vi "SPI_CY_target.vi"() -> ()   [LabVIEW 2018]
uses:
  <vilib>/Platform/TimedLoop/XDataNode/timing_clust.ctl
  <vilib>/Platform/TimedLoop/XDataNode/nitl_modes.ctl
  <vilib>/Platform/TimedLoop/XDataNode/wakeup.ctl
  <vilib>/rvi/Emulation/niFpgaGetClockAttributes.vi
  <vilib>/rvi/Emulation/niFpgaSctlEmulationGetInTimedLoop.vi
  <vilib>/rvi/Emulation/niFpgaEmulationReportErrorSimple.vi
  <vilib>/rvi/eio/common/nirviEmuTemplateMethod_errors.vi
  <vilib>/rvi/Emulation/niFpgaCriticalErrorInLSC.vi
  <vilib>/rvi/Emulation/niFpgaProcessEmulError.vi
  <vilib>/rvi/interface/RandomDataEmulation/niFpgaRandomDataHandleErrors.vi
  <vilib>/eio/EIONode/EIONode.xnode
  <vilib>/Platform/TimedLoop/XDataNode/XDataNode.xnode
  <vilib>/rvi/DataTransferAndStorage/Container/XNode/niFpgaContainer.xnode
  <vilib>/rvi/interface/RandomDataEmulation/nirviRandomDataFpgaReadWriteTemplate.vi
  <vilib>/Platform/TimedLoop/XDataNode/XDNodeRunTimeDep.lvlib
panel:
  out "Addr Read":u32
  out "WriteError":bool
  out "Addr":u32
  out "WriteChipComplete":bool
  in  "i":i32
  in  "Parts":i32
  in  "ReadDelay":u8
  in  "Stop":bool
  in  "ReadWords":u32
  in  "NextPart":bool
  out "ReadChipComplete":bool
  in  "Source Name":refnum<k21>="20MHz"
  in  "SelectOperation":enum16{"Read", "Write"}(ring)
  in  "OperationComplete":bool
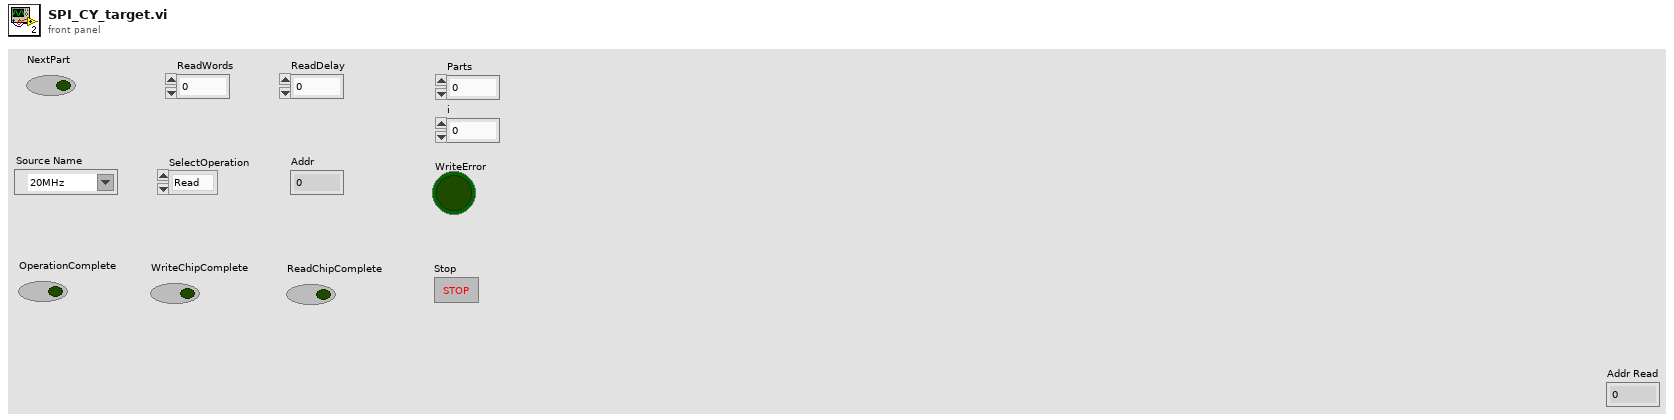
[diagram p1: front panel]
types:
  T1 = typedef "XDNodeRunTimeDep.lvlib/timing_clust.ctl" = cluster{"Expected End [f-1]":u64, "Actual End [f-1]":u64, "Finished Late? [f-1]":bool, "Expected End [i-1]":u64, "Actual End [i-1]":u64, "Finished Late? [i-1]":bool, "Expected Start [i]":u64, "Actual Start [i]":u64, "Expected Start [f]":u64, "Actual Start [f]":u64, "Source Name":string, "Structure Name":string, "Period":i64, "Deadline":i64, "Offset":i64, "Start":i64, "Priority":i32, "Timeout":i32, "Mode":T2, "Wakeup Reason":T3, "Error":errorcluster, "Source Type":string, "Secondary Source Type":string, "Global End Time":u64, "Global Start Time":u64, "Frame Duration":u64, "Iteration Duration":u64, "Assigned CPU":i32, "I/O Scan Engine Mode":u32}
  T2 = typedef "XDNodeRunTimeDep.lvlib/nitl_modes.ctl" = enum32{"No Change", "Process missed periods, maintain original phase", "Discard missed periods, maintain original phase", "Process missed periods, ignore original phase", "Discard missed periods, ignore original phase"}
  T3 = typedef "XDNodeRunTimeDep.lvlib/wakeup.ctl" = enum32{"Normal", "Aborted", "Asynchronous wakeup", "Timing source error", "Timed loop error", "Timeout"}
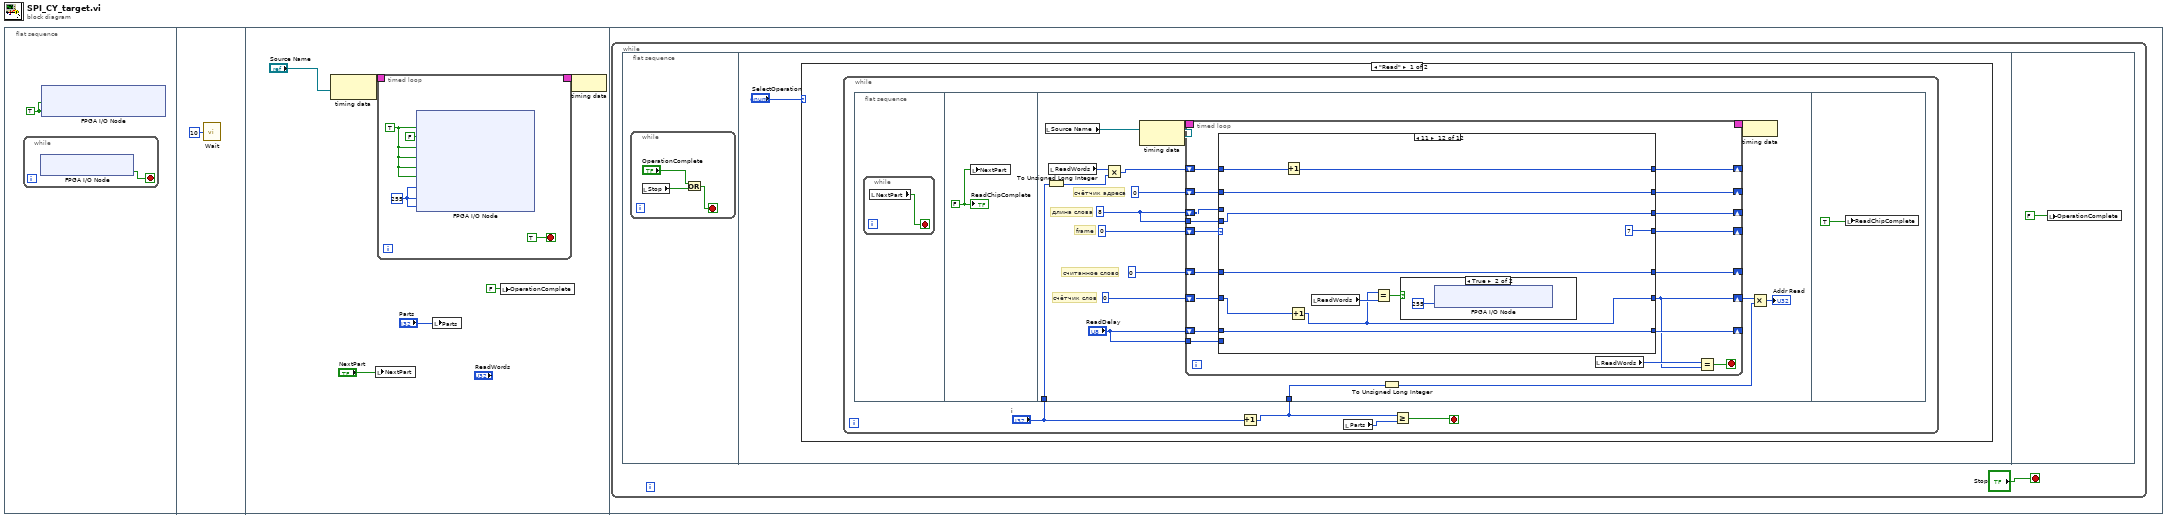
[diagram p0: block diagram]
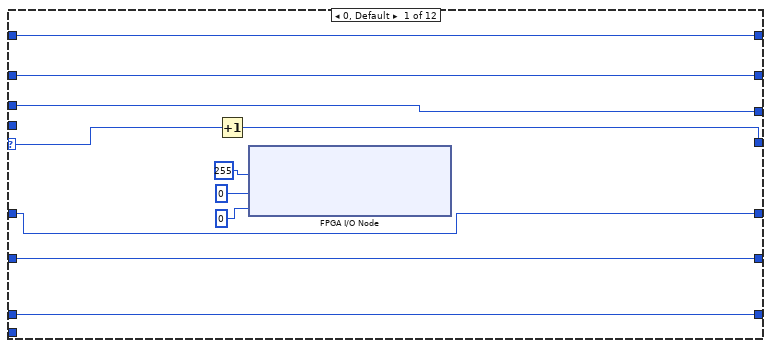
[diagram p2: hidden frame]
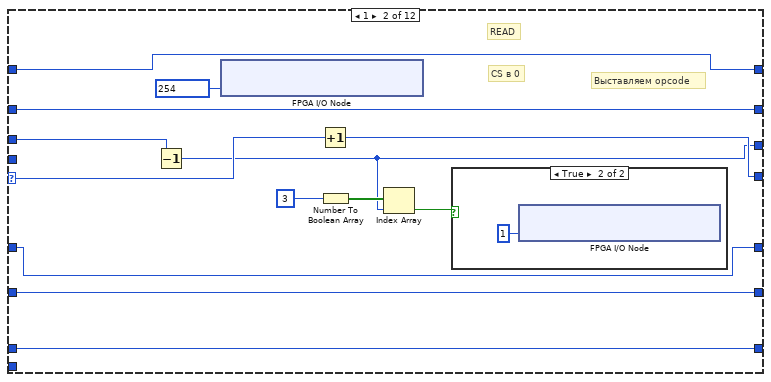
[diagram p3: hidden frame]
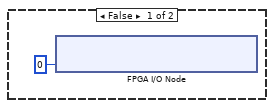
[diagram p4: hidden frame]
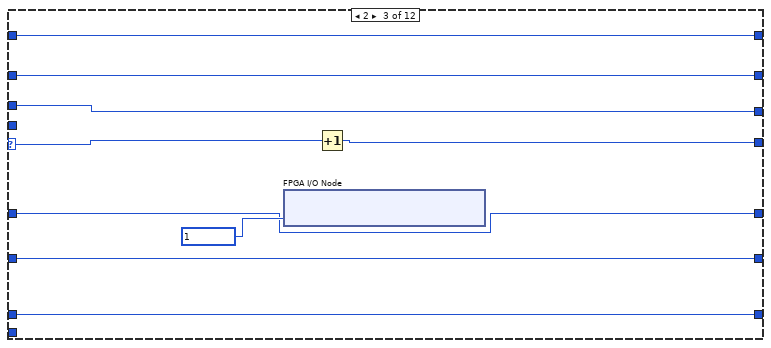
[diagram p5: hidden frame]
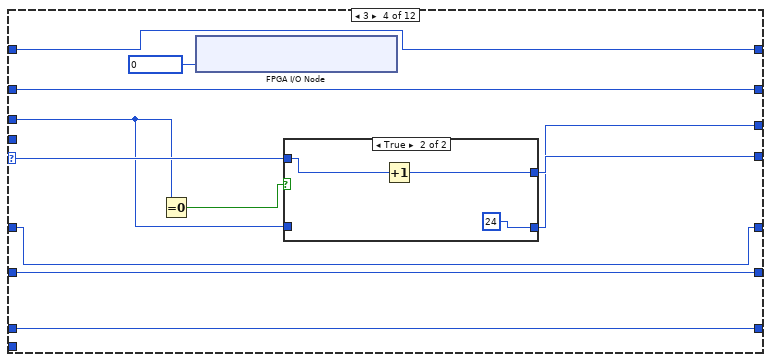
[diagram p6: hidden frame]
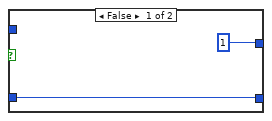
[diagram p7: hidden frame]
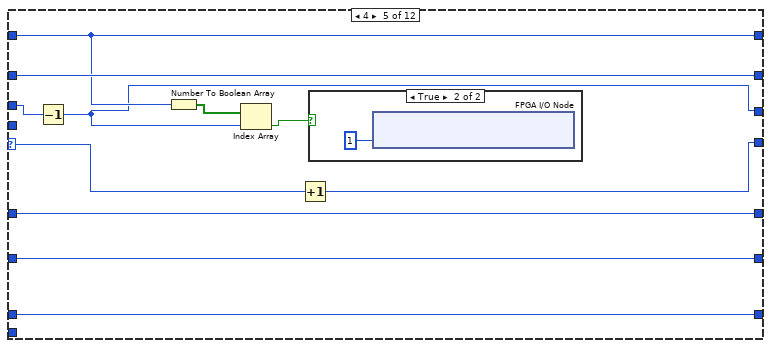
[diagram p8: hidden frame]
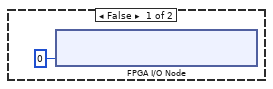
[diagram p9: hidden frame]
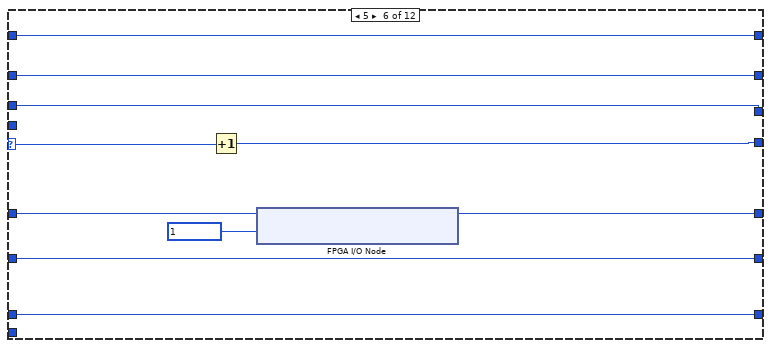
[diagram p10: hidden frame]
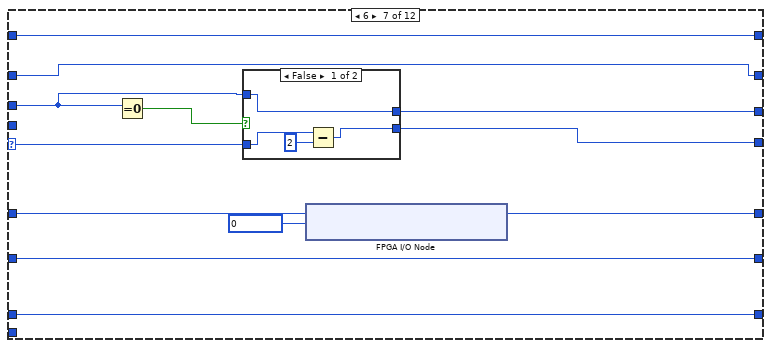
[diagram p11: hidden frame]
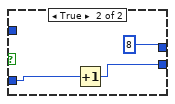
[diagram p12: hidden frame]
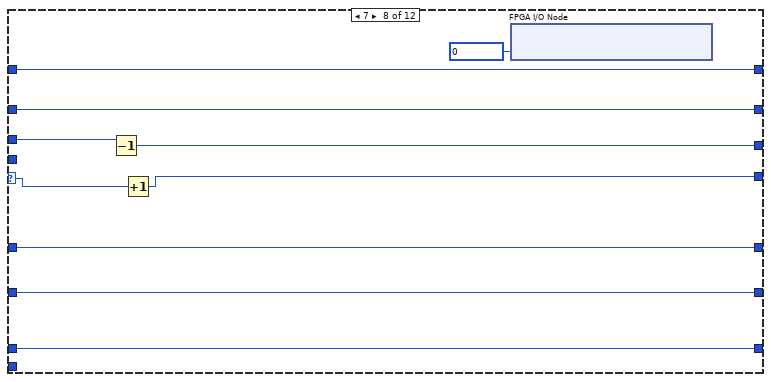
[diagram p13: hidden frame]
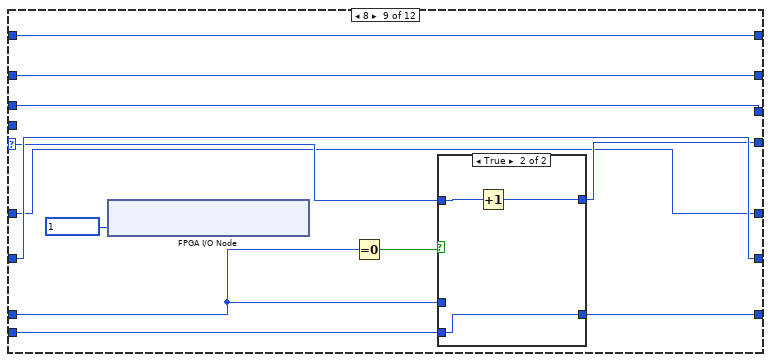
[diagram p14: hidden frame]
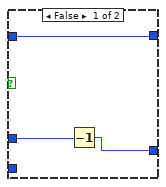
[diagram p15: hidden frame]
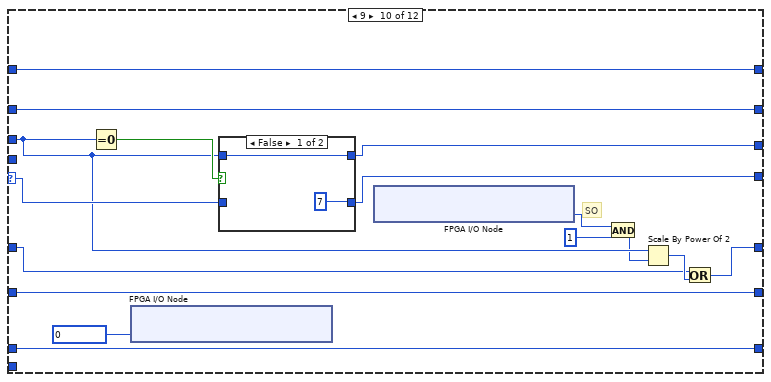
[diagram p16: hidden frame]
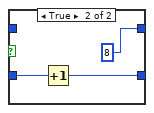
[diagram p17: hidden frame]
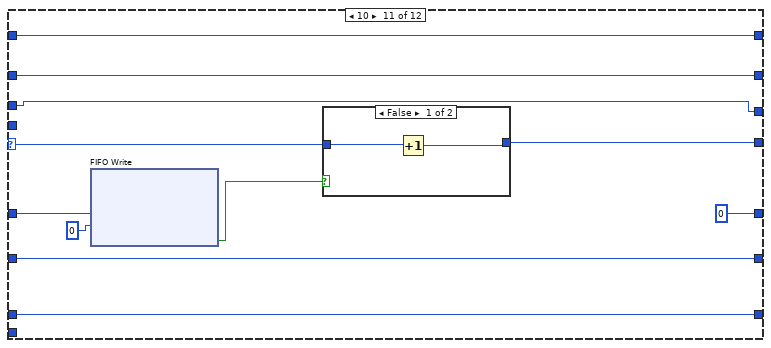
[diagram p18: hidden frame]
diagram:
  n1 = flat-sequence {
    frame #0 {
      w1 = TRUE ("IO Module\\DDCB_Supply_Select")
      n2 = while {
        stop <- w2 stop-if-true
        n3 = xnode "FPGA I/O Node"() -> ("IO Module IO Enabled"=w2:bool)  [unwired: 1 in, 1 out]
      }
      n4 = xnode "FPGA I/O Node"("IO Module\\DDCB_Supply_Select"=w1, "IO Module\\DDCA_Supply_Select"=w1) -> ()  [unwired: 2 in, 2 out]
    }
    frame #1 {
      n5 = call "Wait"("Count(mSec)"=u8 10) -> ()  [unwired: 1 out]
    }
    frame #2 {
      n6 = node-c288("Source Name") -> (w9:T1)
      n7 = local write "NextPart"("NextPart") -> ()
      n8 = timed-loop {
        timing: w9 -> [_]
        timing-out: [_] -> w8
        stop <- TRUE stop-if-true
        w10 = u8 255
        w11 = TRUE ("IO Module\\DDCA_Port1_WE")
        n9 = xnode "FPGA I/O Node"("IO Module\\DDCA_Port0_WE"=w11, "IO Module\\DDCA_Port1_WE"=FALSE ("IO Module\\DDCA_Port1_WE"), "IO Module\\DDCB_Port0_WE"=w11, "IO Module\\DDCB_Port1_WE"=w11, "IO Module\\DDCA_PFI_WE"=w11, "IO Module\\DDCB_PFI_WE"=w11, "IO Module\\DDCA_Port0_Write"=w10, "IO Module\\DDCB_Port0_Write"=w10, "IO Module\\DDCB_Port1_Write"=w10) -> ()  [unwired: 9 in, 9 out]
      }
      n10 = local write "Parts"("Parts") -> ()
      n11 = local write "OperationComplete"(FALSE ("OperationComplete")) -> ()
      n12 = node-c288(w8) -> ()
    }
    frame #3 {
      n13 = while {
        stop <- "Stop" stop-if-true
        n14 = flat-sequence {
          frame #0 {
            n15 = while {
              stop <- w22 stop-if-true
              n16 = local read "Stop"() -> (w21:bool)
              n17 = Or(x="OperationComplete", y=w21) -> (x .or. y?=w22:bool)
            }
          }
          frame #1 {
            n18 = case shown="\"Read\"" "SelectOperation" {
              frame "Read" {
                n19 = while {
                  stop <- w26 stop-if-true
                  n20 = flat-sequence {
                    tunnel: "i" -> [w35]
                    tunnel: w25 -> [w34]
                    frame #0 {
                      n21 = while {
                        stop <- w29 stop-if-true
                        n22 = local read "NextPart"() -> (w29:bool)
                      }
                    }
                    frame #1 {
                      w30 = FALSE ("Boolean")
                      n23 = local write "NextPart"(w30) -> ()
                      "ReadChipComplete" <- w30
                    }
                    frame #2 {
                      w39 = 8
                      # "считанное слово"
                      # "длина слова"
                      # "счётчик адреса"
                      # "frame"
                      # "счётчик слов"
                      n24 = local read "Source Name"() -> (w45:refnum<k21>)
                      n25 = To Unsigned Long Integer(number=w35) -> (unsigned 32bit integer=w36:u32)
                      n26 = local read "ReadWords"() -> (w37:u32)
                      n27 = Multiply(x=w37, y=w36) -> (x*y=w38:u32)
                      n28 = node-c288(w45) -> (w47:T1)
                      n29 = timed-loop {
                        timing: w47 -> [_]
                        timing-out: [_] -> w46
                        shift-right: [w61] -> _
                        shift-left: i16 0 -> [w65]
                        shift-right: [w48] -> w32
                        shift-left: u32 0 -> [w62]
                        shift-right: [w59] -> _
                        shift-left: i16 0 -> [w60]
                        shift-right: [w57] -> _
                        shift-left: w39 -> [w58]
                        shift-right: [w55] -> _
                        shift-left: w38 -> [w56]
                        tunnel: "ReadDelay" -> [w52]
                        shift-right: [w53] -> _
                        shift-left: "ReadDelay" -> [w54]
                        shift-right: [w51] -> _
                        shift-left: u8 0 -> [w50]
                        tunnel: w39 -> [w49]
                        stop <- w63 stop-if-true
                        n30 = case shown="11" w65 {
                          selector: w65 -> [w75 w88 w99 w108 w126 w137 w146 w161 w169 w194 w211 _]
                          tunnel: w62 -> [w76 w89 w95 w110 w127 w132 w148 w159 w176 w198 w215 w228]
                          tunnel: [w76 w89 w95 w110 w127 w132 w148 w159 w176 w198 w215 w220] -> w48
                          tunnel: [w74 w87 w98 w107 w125 w136 w145 w160 w168 w193 w210 i16 7] -> w61
                          tunnel: w60 -> [w70 w86 w97 w111 w124 w134 w141 w165 w177 w195 w208 w230]
                          tunnel: [w70 w86 w97 w111 w124 w134 w141 w165 w177 w195 w208 w230] -> w59
                          tunnel: w58 -> [w69 w85 w96 w106 w120 w135 w144 w163 w174 w191 w206 _]
                          tunnel: [w69 w82 w96 w105 w119 w135 w143 w162 w174 w192 w206 w227] -> w57
                          tunnel: w56 -> [w68 w79 w94 w103 w121 w133 w142 w166 w178 w197 w207 w229]
                          tunnel: [w68 w79 w94 w103 w121 w133 w142 w166 w178 w197 w207 w223] -> w55
                          tunnel: w54 -> [w67 w78 w93 w102 w118 w131 w140 w158 w171 w199 w216 w226]
                          tunnel: [w67 w78 w93 w102 w118 w131 w140 w158 w170 w199 w216 w226] -> w53
                          tunnel: w52 -> [_ _ _ _ _ _ _ _ w172 _ _ _]
                          tunnel: [w66 w77 w92 w101 w117 w130 w139 w157 w167 w186 u8 0 w224] -> w51
                          tunnel: w50 -> [w66 w77 w92 w101 w117 w130 w139 w157 w167 w185 w214 w224]
                          tunnel: w49 -> [_ _ _ _ _ _ _ _ _ _ _ w227]
                          frame 0, Default {
                            n31 = Increment(x=w75) -> (x+1=w74:i16)
                            n32 = xnode "FPGA I/O Node"("IO Module\\DDCA_Port0_Write"=u8 255, "IO Module\\DDCB_Port0_Write"=u8 0 ("IO Module\\DDCB_Port0_Write"), "IO Module\\DDCB_Port1_Write"=u8 0 ("IO Module\\DDCB_Port1_Write")) -> ()  [unwired: 3 in, 3 out]
                          }
                          frame 1 {
                            # "Выставляем opcode"
                            # "CS в 0"
                            # "READ"
                            n33 = Decrement(x=w85) -> (x-1=w82:i32)
                            n34 = xnode "FPGA I/O Node"("IO Module\\DDCA_Port0_Write"=u8 254 ("IO Module\\DDCB_Port1_Write")) -> ()  [unwired: 1 in, 1 out]
                            n35 = Increment(x=w88) -> (x+1=w87:i16)
                            n36 = Number To Boolean Array(number=u8 3) -> (Boolean array=w83:bool[])
                            n37 = Index Array(array=w83, index=w82) -> (element=w81:bool)
                            n38 = case shown="True" w81 {
                              frame False {
                                n39 = xnode "FPGA I/O Node"("IO Module\\DDCB_Port1_Write"=u8 0 ("IO Module\\DDCB_Port1_Write")) -> ()  [unwired: 1 in, 1 out]
                              }
                              frame True {
                                n40 = xnode "FPGA I/O Node"("IO Module\\DDCB_Port1_Write"=u8 1 ("IO Module\\DDCB_Port1_Write")) -> ()  [unwired: 1 in, 1 out]
                              }
                            }
                          }
                          frame 2 {
                            n41 = xnode "FPGA I/O Node"("IO Module\\DDCB_Port0_Write"=u8 1 ("IO Module\\DDCB_Port1_Write")) -> ()  [unwired: 1 in, 1 out]
                            n42 = Increment(x=w99) -> (x+1=w98:i16)
                          }
                          frame 3 {
                            n43 = Equal To 0?(x=w106) -> (x = 0?=w109:bool)
                            n44 = xnode "FPGA I/O Node"("IO Module\\DDCB_Port0_Write"=u8 0 ("IO Module\\DDCB_Port1_Write")) -> ()  [unwired: 1 in, 1 out]
                            n45 = case shown="True" w109 {
                              tunnel: w108 -> [_ w116]
                              tunnel: [i16 1 w115] -> w107
                              tunnel: [w112 24] -> w105
                              tunnel: w106 -> [w112 _]
                              frame False {
                              }
                              frame True {
                                n46 = Increment(x=w116) -> (x+1=w115:i16)
                              }
                            }
                          }
                          frame 4 {
                            n47 = Decrement(x=w120) -> (x-1=w119:i32)
                            n48 = Number To Boolean Array(number=w121) -> (Boolean array=w122:bool[])
                            n49 = Index Array(array=w122, index=w119) -> (element=w123:bool)
                            n50 = Increment(x=w126) -> (x+1=w125:i16)
                            n51 = case shown="True" w123 {
                              frame False {
                                n52 = xnode "FPGA I/O Node"("IO Module\\DDCB_Port1_Write"=u8 0 ("IO Module\\DDCB_Port1_Write")) -> ()  [unwired: 1 in, 1 out]
                              }
                              frame True {
                                n53 = xnode "FPGA I/O Node"("IO Module\\DDCB_Port1_Write"=u8 1 ("IO Module\\DDCB_Port1_Write")) -> ()  [unwired: 1 in, 1 out]
                              }
                            }
                          }
                          frame 5 {
                            n54 = Increment(x=w137) -> (x+1=w136:i16)
                            n55 = xnode "FPGA I/O Node"("IO Module\\DDCB_Port0_Write"=u8 1 ("IO Module\\DDCB_Port1_Write")) -> ()  [unwired: 1 in, 1 out]
                          }
                          frame 6 {
                            n56 = Equal To 0?(x=w144) -> (x = 0?=w147:bool)
                            n57 = case shown="False" w147 {
                              tunnel: w146 -> [w153 w156]
                              tunnel: [w151 w155] -> w145
                              tunnel: w144 -> [w150 _]
                              tunnel: [w150 8] -> w143
                              frame False {
                                n58 = Subtract(x=w153, y=i16 2) -> (x-y=w151:i16)
                              }
                              frame True {
                                n59 = Increment(x=w156) -> (x+1=w155:i16)
                              }
                            }
                            n60 = xnode "FPGA I/O Node"("IO Module\\DDCB_Port0_Write"=u8 0 ("IO Module\\DDCB_Port1_Write")) -> ()  [unwired: 1 in, 1 out]
                          }
                          frame 7 {
                            n61 = Decrement(x=w163) -> (x-1=w162:i32)
                            n62 = Increment(x=w161) -> (x+1=w160:i16)
                            n63 = xnode "FPGA I/O Node"("IO Module\\DDCB_Port0_Write"=u8 0 ("IO Module\\DDCB_Port1_Write")) -> ()  [unwired: 1 in, 1 out]
                          }
                          frame 8 {
                            n64 = xnode "FPGA I/O Node"("IO Module\\DDCB_Port0_Write"=u8 1 ("IO Module\\DDCB_Port1_Write")) -> ()  [unwired: 1 in, 1 out]
                            n65 = Equal To 0?(x=w171) -> (x = 0?=w173:bool)
                            n66 = case shown="True" w173 {
                              tunnel: w172 -> [_ w184]
                              tunnel: w171 -> [w181 _]
                              tunnel: [w180 w184] -> w170
                              tunnel: w169 -> [w179 w183]
                              tunnel: [w179 w182] -> w168
                              frame False {
                                n67 = Decrement(x=w181) -> (x-1=w180:u8)
                              }
                              frame True {
                                n68 = Increment(x=w183) -> (x+1=w182:i16)
                              }
                            }
                          }
                          frame 9 {
                            # "SO"
                            n69 = Equal To 0?(x=w191) -> (x = 0?=w196:bool)
                            n70 = xnode "FPGA I/O Node"("IO Module\\DDCB_Port0_Write"=u8 0 ("IO Module\\DDCB_Port1_Write")) -> ()  [unwired: 1 in, 1 out]
                            n71 = case shown="False" w196 {
                              tunnel: w194 -> [_ w205]
                              tunnel: [i16 7 w204] -> w193
                              tunnel: [w201 8] -> w192
                              tunnel: w191 -> [w201 _]
                              frame False {
                              }
                              frame True {
                                n72 = Increment(x=w205) -> (x+1=w204:i16)
                              }
                            }
                            n73 = xnode "FPGA I/O Node"() -> ("IO Module\\DDCA_Port1_Read"=w188:u8)  [unwired: 1 in, 1 out]
                            n74 = And(x=w188, y=u8 1) -> (x .and. y?=w190:u8)
                            n75 = Scale By Power Of 2(n=w191, x=w190) -> (x*2^n=w187:u8)
                            n76 = Or(x=w185, y=w187) -> (x .or. y?=w186:u8)
                          }
                          frame 10 {
                            n77 = xnode ("FIFO Write")("Element"=w214, "Timeout"=0) -> ("Timed Out?"=w212:bool)  [unwired: 1 in, 1 out]
                            n78 = case shown="False" w212 {
                              tunnel: w211 -> [w217 w219]
                              tunnel: [w218 w219] -> w210
                              frame False {
                                n79 = Increment(x=w217) -> (x+1=w218:i16)
                              }
                              frame True {
                              }
                            }
                          }
                          frame 11 {
                            n80 = Increment(x=w229) -> (x+1=w223:u32)
                            n81 = Increment(x=w228) -> (x+1=w220:u32)
                            n82 = local read "ReadWords"() -> (w222:u32)
                            n83 = Equal?(x=w220, y=w222) -> (x = y?=w221:bool)
                            n84 = case shown="True" w221 {
                              frame False {
                              }
                              frame True {
                                n85 = xnode "FPGA I/O Node"("IO Module\\DDCA_Port0_Write"=u8 255 ("IO Module\\DDCA_Port0_Write")) -> ()  [unwired: 1 in, 1 out]
                              }
                            }
                          }
                        }
                        n86 = local read "ReadWords"() -> (w64:u32)
                        n87 = Equal?(x=w64, y=w48) -> (x = y?=w63:bool)
                      }
                      n88 = To Unsigned Long Integer(number=w34) -> (unsigned 32bit integer=w31:u32)
                      n89 = node-c288(w46) -> ()
                      n90 = Multiply(x=w32, y=w31) -> (x*y=→"Addr Read":u32)
                    }
                    frame #3 {
                      n91 = local write "ReadChipComplete"(TRUE ("ReadChipComplete")) -> ()
                    }
                  }
                  n92 = Increment(x="i") -> (x+1=w25:i32)
                  n93 = local read "Parts"() -> (w28:i32)
                  n94 = Greater Or Equal?(x=w25, y=w28) -> (x >= y?=w26:bool)
                }
              }
              frame "Write" {
                n95 = while {
                  i -> [w239]
                  stop <- w240 stop-if-true
                  # "32 части (всего)"
                  n96 = flat-sequence {
                    tunnel: w239 -> [w248]
                    frame #0 {
                      n97 = while {
                        stop <- w243 stop-if-true
                        n98 = local read "NextPart"() -> (w243:bool)
                      }
                    }
                    frame #1 {
                      w244 = FALSE ("WriteChipComplete")
                      n99 = local write "NextPart"(w244) -> ()
                      "WriteChipComplete" <- w244
                    }
                    frame #2 {
                      # "error write"
                      # "счетчик записанных слов"
                      # "записанное значение"
                      # "counter"
                      n100 = local read "Source Name"() -> (w255:refnum<k21>)
                      n101 = To Unsigned Long Integer(number=w248) -> (unsigned 32bit integer=w249:u32)
                      n102 = node-c288(w255) -> (w257:T1)
                      n103 = Multiply(x=u32 65536, y=w249) -> (x*y=w250:u32)
                      n104 = timed-loop {
                        timing: w257 -> [_]
                        timing-out: [_] -> w256
                        shift-right: [w273] -> _
                        shift-left: 8 -> [w276]
                        shift-right: [w274] -> _
                        shift-left: 0 -> [w275]
                        shift-right: [w268] -> _
                        shift-left: u8 0 -> [w269]
                        shift-right: [w270] -> _
                        shift-left: u16 0 -> [w271]
                        shift-right: [w258] -> _
                        shift-left: i64 0 -> [w272]
                        shift-right: [w266] -> _
                        shift-left: w250 -> [w267]
                        shift-right: [w263] -> _
                        shift-left: u32 0 -> [w265]
                        stop <- w262 stop-if-true
                        n105 = case shown="14" w275 {
                          selector: w275 -> [w284 w295 w308 w320 w336 w351 w360 w373 w386 w397 w412 w424 w439 w447 w464 w481 w489 w503 w515 w531 w540 w545 w565 w574 _]
                          tunnel: w276 -> [w282 w298 w309 w316 w337 w348 w354 w378 w387 w394 w413 w428 w437 w445 w467 w479 w493 w504 w511 w529 w538 w543 w563 w572 w592]
                          tunnel: [w283 w294 w307 w319 w335 w349 w359 w372 w385 w396 w411 w423 w438 w446 w458 w480 w488 w502 w514 w530 w539 w544 w564 w573 0] -> w274
                          tunnel: [w282 w289 w309 w318 w331 w348 w358 w374 w387 w395 w413 w425 w437 w448 w467 w479 w487 w504 w513 w528 w538 w542 w563 w572 w592] -> w273
                          tunnel: w272 -> [w281 w290 w304 w313 w332 w345 w357 w371 w382 w391 w407 w420 w434 w442 w460 w475 w486 w499 w510 w526 w534 w549 w559 w568 w588]
                          tunnel: [w281 w290 w304 w313 w332 w345 w357 w371 w382 w391 w407 w420 w434 w442 w460 w475 w486 w499 w510 w526 w534 w549 w559 w567 w588] -> w258
                          tunnel: w271 -> [w280 w291 w305 w314 w333 w346 w356 w370 w383 w392 w408 w421 w435 w443 w466 w476 w485 w500 w509 w525 w535 w548 w560 w569 w589]
                          tunnel: [w280 w291 w305 w314 w333 w346 w356 w370 w383 w392 w408 w421 w435 w443 w459 w476 w485 w500 w509 w525 w535 w548 w560 w569 w589] -> w270
                          tunnel: w269 -> [w279 w292 w306 w315 w334 w347 w355 w369 w384 w393 _ w422 w436 w444 w461 w477 w484 w501 w508 w524 w536 w547 w561 w570 w590]
                          tunnel: [w279 w292 w306 w315 w334 w347 w355 w369 w384 w393 w409 w422 w436 w444 w461 w477 w484 w501 w508 w524 w536 w547 w561 w570 w590] -> w268
                          tunnel: w267 -> [w278 w288 w303 w312 w330 w344 w353 w376 w388 w398 w414 w429 w440 w450 w468 w478 w494 w505 w512 w527 w537 w552 w562 w576 w595]
                          tunnel: [w278 w288 w303 w312 w330 w344 w353 w376 w388 w398 w414 w429 w440 w450 w468 w478 w494 w505 w512 w527 w537 w552 w562 w576 w593] -> w266
                          tunnel: w265 -> [w277 w287 w302 w311 w328 w343 w352 w368 w381 w390 w406 w419 w432 w441 w457 w474 w483 w498 w507 w523 w533 w550 w558 w571 w598]
                          tunnel: [w277 w287 w302 w311 w328 w343 w352 w368 w381 w390 w406 w419 w432 w441 w457 w474 w483 w498 w507 w523 w533 w550 w558 w571 w597] -> w263
                          frame 0, Default {
                            w285 = u8 0 ("IO Module\\DDCB_Port0_Write")
                            n106 = xnode "FPGA I/O Node"("IO Module\\DDCA_Port0_Write"=u8 255 ("IO Module\\DDCA_Port0_Write"), "IO Module\\DDCB_Port0_Write"=w285, "IO Module\\DDCB_Port1_Write"=w285) -> ()  [unwired: 3 in, 3 out]
                            n107 = Increment(x=w284) -> (x+1=w283:i32)
                          }
                          frame 1 {
                            n108 = xnode "FPGA I/O Node"("IO Module\\DDCA_Port0_Write"=u8 254 ("IO Module\\DDCA_Port0_Write")) -> ()  [unwired: 1 in, 1 out]
                            n109 = Decrement(x=w298) -> (x-1=w289:i32)
                            n110 = Number To Boolean Array(number=u8 6) -> (Boolean array=w297:bool[])
                            n111 = Index Array(array=w297, index=w289) -> (element=w299:bool)
                            n112 = Increment(x=w295) -> (x+1=w294:i32)
                            n113 = case shown="False" w299 {
                              frame False {
                                n114 = xnode "FPGA I/O Node"("IO Module\\DDCB_Port1_Write"=u8 0 ("IO Module\\DDCB_Port1_Write")) -> ()  [unwired: 1 in, 1 out]
                              }
                              frame True {
                                n115 = xnode "FPGA I/O Node"("IO Module\\DDCB_Port1_Write"=u8 1 ("IO Module\\DDCB_Port1_Write")) -> ()  [unwired: 1 in, 1 out]
                              }
                            }
                          }
                          frame 2 {
                            n116 = Increment(x=w308) -> (x+1=w307:i32)
                            n117 = xnode "FPGA I/O Node"("IO Module\\DDCB_Port0_Write"=u8 1 ("IO Module\\DDCB_Port1_Write")) -> ()  [unwired: 1 in, 1 out]
                          }
                          frame 3 {
                            n118 = xnode "FPGA I/O Node"("IO Module\\DDCB_Port0_Write"=u8 0 ("IO Module\\DDCB_Port1_Write")) -> ()  [unwired: 1 in, 1 out]
                            n119 = Equal To 0?(x=w316) -> (x = 0?=w317:bool)
                            n120 = case shown="True" w317 {
                              tunnel: w320 -> [_ w327]
                              tunnel: [1 w326] -> w319
                              tunnel: [w322 8] -> w318
                              tunnel: w316 -> [w322 _]
                              frame False {
                              }
                              frame True {
                                n121 = Increment(x=w327) -> (x+1=w326:i32)
                                n122 = xnode "FPGA I/O Node"("IO Module\\DDCA_Port0_Write"=u8 255 ("IO Module\\DDCA_Port0_Write")) -> ()  [unwired: 1 in, 1 out]
                              }
                            }
                          }
                          frame 4 {
                            n123 = Decrement(x=w337) -> (x-1=w331:i32)
                            n124 = xnode "FPGA I/O Node"("IO Module\\DDCA_Port0_Write"=u8 254 ("IO Module\\DDCA_Port0_Write")) -> ()  [unwired: 1 in, 1 out]
                            n125 = Number To Boolean Array(number=u8 2) -> (Boolean array=w339:bool[])
                            n126 = Index Array(array=w339, index=w331) -> (element=w340:bool)
                            n127 = Increment(x=w336) -> (x+1=w335:i32)
                            n128 = case shown="False" w340 {
                              frame False {
                                n129 = xnode "FPGA I/O Node"("IO Module\\DDCB_Port1_Write"=u8 0 ("IO Module\\DDCB_Port1_Write")) -> ()  [unwired: 1 in, 1 out]
                              }
                              frame True {
                                n130 = xnode "FPGA I/O Node"("IO Module\\DDCB_Port1_Write"=u8 1 ("IO Module\\DDCB_Port1_Write")) -> ()  [unwired: 1 in, 1 out]
                              }
                            }
                          }
                          frame 5 {
                            n131 = xnode "FPGA I/O Node"("IO Module\\DDCB_Port0_Write"=u8 1 ("IO Module\\DDCB_Port1_Write")) -> ()  [unwired: 1 in, 1 out]
                            n132 = Increment(x=w351) -> (x+1=w349:i32)
                          }
                          frame 6 {
                            n133 = xnode "FPGA I/O Node"("IO Module\\DDCB_Port0_Write"=u8 0 ("IO Module\\DDCB_Port1_Write")) -> ()  [unwired: 1 in, 1 out]
                            n134 = Equal To 0?(x=w354) -> (x = 0?=w361:bool)
                            n135 = case shown="True" w361 {
                              tunnel: w360 -> [_ w367]
                              tunnel: [4 w366] -> w359
                              tunnel: [w364 24] -> w358
                              tunnel: w354 -> [w364 _]
                              frame False {
                              }
                              frame True {
                                # "адресс"
                                n136 = Increment(x=w367) -> (x+1=w366:i32)
                              }
                            }
                          }
                          frame 7 {
                            n137 = Decrement(x=w378) -> (x-1=w374:i32)
                            n138 = Number To Boolean Array(number=w376) -> (Boolean array=w377:bool[])
                            n139 = Index Array(array=w377, index=w374) -> (element=w375:bool)
                            n140 = Increment(x=w373) -> (x+1=w372:i32)
                            n141 = case shown="False" w375 {
                              frame False {
                                n142 = xnode "FPGA I/O Node"("IO Module\\DDCB_Port1_Write"=u8 0 ("IO Module\\DDCB_Port1_Write")) -> ()  [unwired: 1 in, 1 out]
                              }
                              frame True {
                                n143 = xnode "FPGA I/O Node"("IO Module\\DDCB_Port1_Write"=u8 1 ("IO Module\\DDCB_Port1_Write")) -> ()  [unwired: 1 in, 1 out]
                              }
                            }
                          }
                          frame 8 {
                            n144 = xnode "FPGA I/O Node"("IO Module\\DDCB_Port0_Write"=u8 1 ("IO Module\\DDCB_Port1_Write")) -> ()  [unwired: 1 in, 1 out]
                            n145 = Increment(x=w386) -> (x+1=w385:i32)
                          }
                          frame 9 {
                            n146 = Equal To 0?(x=w394) -> (x = 0?=w399:bool)
                            n147 = xnode "FPGA I/O Node"("IO Module\\DDCB_Port0_Write"=u8 0 ("IO Module\\DDCB_Port1_Write")) -> ()  [unwired: 1 in, 1 out]
                            n148 = case shown="True" w399 {
                              tunnel: w397 -> [_ w405]
                              tunnel: [7 w404] -> w396
                              tunnel: [w402 8] -> w395
                              tunnel: w394 -> [w402 _]
                              frame False {
                              }
                              frame True {
                                n149 = Increment(x=w405) -> (x+1=w404:i32)
                              }
                            }
                          }
                          frame 10 {
                            n150 = xnode ("FIFO Method Node")("Timeout"=0) -> ("Element"=w409:u8, "Timed Out?"=w410:bool)  [unwired: 1 in, 1 out]
                            n151 = case shown="False" w410 {
                              tunnel: w412 -> [w417 w418]
                              tunnel: [w416 w418] -> w411
                              frame False {
                                n152 = Increment(x=w417) -> (x+1=w416:i32)
                              }
                              frame True {
                              }
                            }
                          }
                          frame 11 {
                            # "Запись значения по адресу (значение получаем из хоста)"
                            n153 = Decrement(x=w428) -> (x-1=w425:i32)
                            n154 = Number To Boolean Array(number=w422) -> (Boolean array=w426:bool[])
                            n155 = Index Array(array=w426, index=w425) -> (element=w427:bool)
                            n156 = Increment(x=w424) -> (x+1=w423:i32)
                            n157 = case shown="False" w427 {
                              frame False {
                                n158 = xnode "FPGA I/O Node"("IO Module\\DDCB_Port1_Write"=u8 0 ("IO Module\\DDCB_Port1_Write")) -> ()  [unwired: 1 in, 1 out]
                              }
                              frame True {
                                n159 = xnode "FPGA I/O Node"("IO Module\\DDCB_Port1_Write"=u8 1 ("IO Module\\DDCB_Port1_Write")) -> ()  [unwired: 1 in, 1 out]
                              }
                            }
                          }
                          frame 12 {
                            n160 = xnode "FPGA I/O Node"("IO Module\\DDCB_Port0_Write"=u8 1 ("IO Module\\DDCB_Port1_Write")) -> ()  [unwired: 1 in, 1 out]
                            n161 = Increment(x=w439) -> (x+1=w438:i32)
                          }
                          frame 13 {
                            n162 = Equal To 0?(x=w445) -> (x = 0?=w449:bool)
                            n163 = xnode "FPGA I/O Node"("IO Module\\DDCB_Port0_Write"=u8 0 ("IO Module\\DDCB_Port1_Write")) -> ()  [unwired: 1 in, 1 out]
                            n164 = case shown="True" w449 {
                              tunnel: [w452 8] -> w448
                              tunnel: w447 -> [_ w455]
                              tunnel: [11 w454] -> w446
                              tunnel: w445 -> [w452 _]
                              frame False {
                              }
                              frame True {
                                n165 = Increment(x=w455) -> (x+1=w454:i32)
                              }
                            }
                          }
                          frame 14 {
                            n166 = Increment(x=w466) -> (x+1=w462:u16)
                            n167 = Equal?(x=w462, y=u16 256) -> (x = y?=w463:bool)
                            n168 = case shown="False" w463 {
                              tunnel: w464 -> [_ w473]
                              tunnel: [10 w472] -> w458
                              tunnel: w462 -> [w469 _]
                              tunnel: [w469 u16 0] -> w459
                              frame False {
                              }
                              frame True {
                                n169 = Increment(x=w473) -> (x+1=w472:i32)
                              }
                            }
                          }
                          frame 15 {
                            n170 = Increment(x=w481) -> (x+1=w480:i32)
                            n171 = xnode "FPGA I/O Node"("IO Module\\DDCA_Port0_Write"=u8 255 ("IO Module\\DDCA_Port0_Write")) -> ()  [unwired: 1 in, 1 out]
                          }
                          frame 16 {
                            # "RDSR"
                            n172 = Decrement(x=w493) -> (x-1=w487:i32)
                            n173 = xnode "FPGA I/O Node"("IO Module\\DDCA_Port0_Write"=u8 254 ("IO Module\\DDCA_Port0_Write")) -> ()  [unwired: 1 in, 1 out]
                            n174 = Number To Boolean Array(number=u8 5) -> (Boolean array=w491:bool[])
                            n175 = Index Array(array=w491, index=w487) -> (element=w490:bool)
                            n176 = Increment(x=w489) -> (x+1=w488:i32)
                            n177 = case shown="True" w490 {
                              frame False {
                                n178 = xnode "FPGA I/O Node"("IO Module\\DDCB_Port1_Write"=u8 0 ("IO Module\\DDCB_Port1_Write")) -> ()  [unwired: 1 in, 1 out]
                              }
                              frame True {
                                n179 = xnode "FPGA I/O Node"("IO Module\\DDCB_Port1_Write"=u8 1 ("IO Module\\DDCB_Port1_Write")) -> ()  [unwired: 1 in, 1 out]
                              }
                            }
                          }
                          frame 17 {
                            n180 = Increment(x=w503) -> (x+1=w502:i32)
                            n181 = xnode "FPGA I/O Node"("IO Module\\DDCB_Port0_Write"=u8 1 ("IO Module\\DDCB_Port1_Write")) -> ()  [unwired: 1 in, 1 out]
                          }
                          frame 18 {
                            n182 = Equal To 0?(x=w511) -> (x = 0?=w516:bool)
                            n183 = xnode "FPGA I/O Node"("IO Module\\DDCB_Port0_Write"=u8 0 ("IO Module\\DDCB_Port1_Write")) -> ()  [unwired: 1 in, 1 out]
                            n184 = case shown="False" w516 {
                              tunnel: w515 -> [_ w522]
                              tunnel: [16 w521] -> w514
                              tunnel: [w518 8] -> w513
                              tunnel: w511 -> [w518 _]
                              frame False {
                              }
                              frame True {
                                n185 = Increment(x=w522) -> (x+1=w521:i32)
                              }
                            }
                          }
                          frame 19 {
                            n186 = xnode "FPGA I/O Node"("IO Module\\DDCB_Port0_Write"=u8 0 ("IO Module\\DDCB_Port1_Write")) -> ()  [unwired: 1 in, 1 out]
                            n187 = Increment(x=w531) -> (x+1=w530:i32)
                            n188 = Decrement(x=w529) -> (x-1=w528:i32)
                          }
                          frame 20 {
                            n189 = xnode "FPGA I/O Node"("IO Module\\DDCB_Port0_Write"=u8 1 ("IO Module\\DDCB_Port1_Write")) -> ()  [unwired: 1 in, 1 out]
                            n190 = Increment(x=w540) -> (x+1=w539:i32)
                          }
                          frame 21 {
                            n191 = Equal To 0?(x=w543) -> (x = 0?=w546:bool)
                            n192 = xnode "FPGA I/O Node"("IO Module\\DDCB_Port0_Write"=u8 0 ("IO Module\\DDCB_Port0_Write")) -> ()  [unwired: 1 in, 1 out]
                            n193 = case shown="True" w546 {
                              tunnel: w545 -> [_ w557]
                              tunnel: [19 w556] -> w544
                              tunnel: w543 -> [w553 _]
                              tunnel: [w553 8] -> w542
                              frame False {
                              }
                              frame True {
                                n194 = Increment(x=w557) -> (x+1=w556:i32)
                              }
                            }
                          }
                          frame 22 {
                            n195 = Increment(x=w565) -> (x+1=w564:i32)
                            n196 = xnode "FPGA I/O Node"("IO Module\\DDCA_Port0_Write"=u8 255 ("IO Module\\DDCA_Port0_Write")) -> ()  [unwired: 1 in, 1 out]
                          }
                          frame 23 {
                            # "SO"
                            n197 = xnode "FPGA I/O Node"() -> ("IO Module\\DDCA_Port1_Read"=w581:u8)  [unwired: 1 in, 1 out]
                            n198 = Number To Boolean Array(number=w581) -> (Boolean array=w579:bool[])
                            n199 = Index Array(array=w579, index=0) -> (element=w577:bool)
                            n200 = And(x=w577, y=TRUE) -> (x .and. y?=w575:bool)
                            n201 = case shown="False" w575 {
                              tunnel: w574 -> [w584 _]
                              tunnel: [w583 16] -> w573
                              tunnel: w568 -> [_ w586]
                              tunnel: [i64 0 w585] -> w567
                              frame False {
                                n202 = Increment(x=w584) -> (x+1=w583:i32)
                              }
                              frame True {
                                n203 = Increment(x=w586) -> (x+1=w585:i64)
                              }
                            }
                          }
                          frame 24 {
                            n204 = Add(x=w598, y=u32 256) -> (x+y=w597:u32)
                            n205 = Add(x=w595, y=u32 256) -> (x+y=w593:u32)
                          }
                        }
                        "Addr" <- w266
                        n206 = Greater Or Equal?(x=w258, y=i64 10000000) -> (x >= y?=w260:bool)
                        "WriteError" <- w260
                        n207 = Equal?(x=w263, y=u32 65536) -> (x = y?=w261:bool)
                        n208 = Or(x=w260, y=w261) -> (x .or. y?=w262:bool)
                      }
                      n209 = node-c288(w256) -> ()
                    }
                    frame #3 {
                      n210 = local write "WriteChipComplete"(TRUE ("WriteChipComplete")) -> ()
                    }
                  }
                  n211 = Increment(x=w239) -> (x+1=w241:i32)
                  n212 = local read "Parts"() -> (w242:i32)
                  n213 = Greater Or Equal?(x=w241, y=w242) -> (x >= y?=w240:bool)
                }
              }
            }
          }
          frame #2 {
            n214 = local write "OperationComplete"(FALSE ("Cycle")) -> ()
          }
        }
      }
    }
  }
